vi "pp2_shock_mA2V.vi"(11 "Shock (mA)":dbl=1000.0) -> (3 "Shock (V)":dbl=0.5)   [LabVIEW 2013]
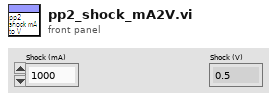
[diagram p1: front panel]
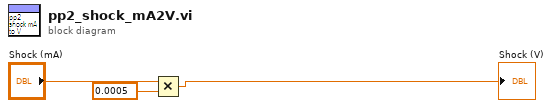
[diagram p0: block diagram]
diagram:
  n1 = Multiply(x="Shock (mA)", y=0.0005) -> (x*y=→"Shock (V)":dbl)
